vi "NetDifference.vi"() -> ()   [LabVIEW 2020]
uses:
  Globals and TypeDefs/Type Definitions.llb/FilePathParameter.ctt
  File and save/X-Axis_Generator_morph.vi
panel:
  out "Exp Index":u32
  in  "AutoSaveData":bool
  in  "stop 2":bool
  in  "SetDirectory?":bool
  in  "FilePath_C":T1={"Filename Prefix"="MyData", "Extension"=enum."±Field", "Suffix"="", "Current Path"=path "/opticsdata/Users"}
  out "?":T2(graph)
  in  "Toggle Subtraction":enum16{"Positive", "Negative"}(ring)
  in  "stop":bool
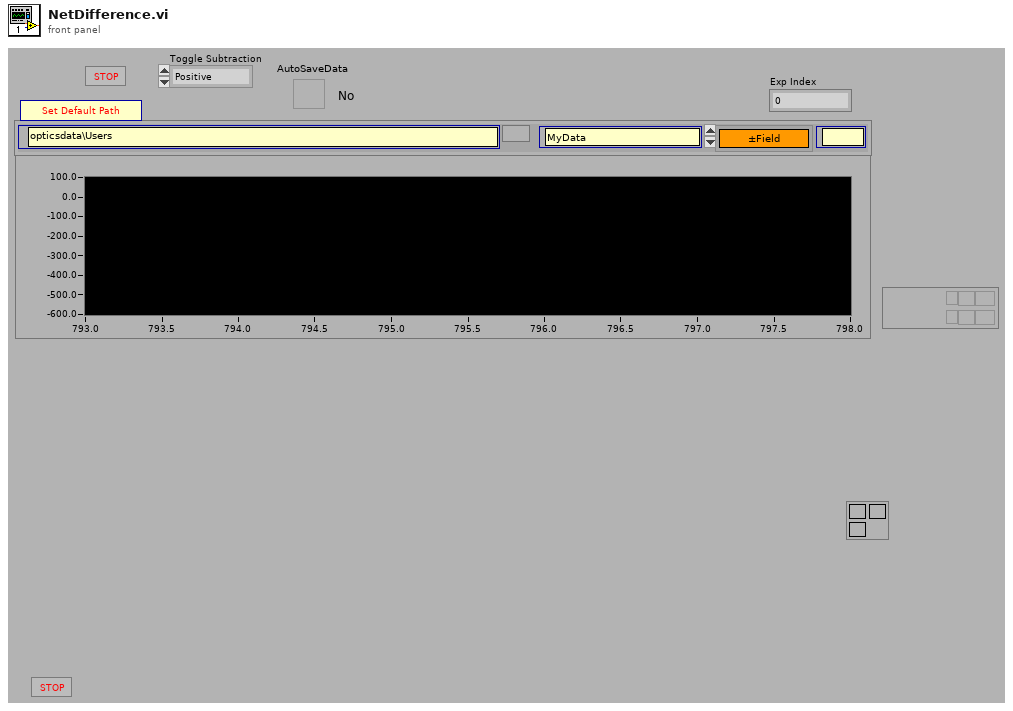
[diagram p1: front panel]
types:
  T1 = typedef "FilePathParameter.ctt" = cluster{"Filename Prefix":string, "Extension":enum16{"none", "\".001\",\".002\", ...", "001 (No dot)", "±Field", "pField nField", "Temperature", "Wavelength", "T(K)±H(T)", "(nm)T(K)±H(T)", "User Defined"}, "Suffix":string, "Current Path":path}
  T2 = cluster{"Ramp Pattern":dbl[], "Sinc Pattern":dbl[]}
  T3 = enum16{"Pass", "Write", "Read", "ReadPlotBlock", "Initialize", "InitFromBufferInput", "Resize Buffer"}
  T4 = enum16{"Auto Data Saving", "Manual Data Saving", "Auto Sequence Saving", "Sequence Saving from Data Buffer"}
  T5 = typedef "FileInfoParameter.ctt" = cluster{"FilePath":path, "Field (T)":dbl, "Temperature (K)":dbl, "X-Axis":T6, "Center nm":dbl, "Current Grating Density":T7, "CCD Parameters":T8, "Operation Mode":T9, "Exp Index":u32, "Index_repetition":u16, "Index":u16, "Current Detector":T10}
  T6 = typedef "Wavelength Unit.ctt" = enum8{"Point", "nm", "eV", "meV", "cm_1"}
  T7 = typedef "McPherson Grating Density.ctl" = enum8{"150", "300", "600", "1200", "1800"}
  T8 = typedef "CCDParameter.ctt" = cluster{"Exposure Time (s)":dbl, "Offset":dbl, "BkgrdCrct":bool, "Shutter":bool, "Mode":enum8{"Regular", "OverExp Cor", "SpikeRemove", "ForCalibration"}, "Repetition":u16, "dt or s":dbl}
  T9 = typedef "OperationMode.ctt" = enum16{"Standby", "CCD Single Shot", "CCD Sequence Shots", "CCD Custom Shots", "CCD Reference Shot", "Step Scanning ", "Time Scanning", "NML Data Acquisition"}
  T10 = typedef "ListOfDetectors.ctt" = enum8{"CCD-1024x256", "InGaAs PDA-1024x1", "CCD-1340x400", "Ge Single Channel", "Si Single Channel", "PMT Single Channel"}
  T11 = enum32{"existing file", "new file", "new or existing file", "existing dir", "new dir", "new or existing dir", "existing file (use LLBs)", "new file (use LLBs)", "new or existing file (use LLBs)", "new or existing file or directory (use LLBs)"}
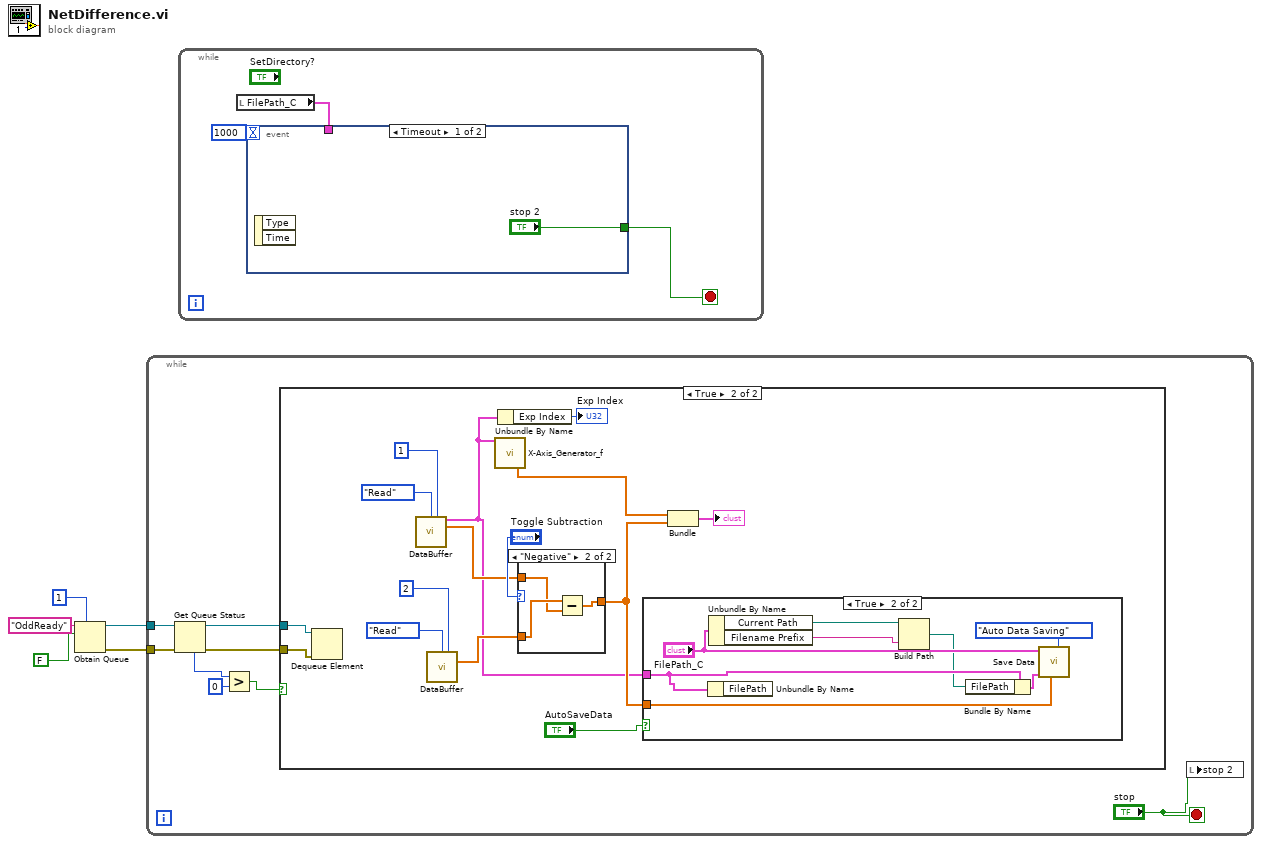
[diagram p0: block diagram]
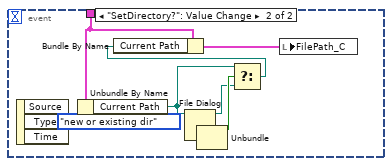
[diagram p2: hidden frame]
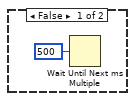
[diagram p3: hidden frame]
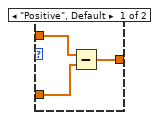
[diagram p5: hidden frame]
diagram:
  n1 = Obtain Queue(max queue size (-1, unlimited)=1, name (unnamed)="OddReady", element data type=FALSE ("Boolean")) -> (queue out=w3:refnum<queue>, error out=w2:errorcluster)  [unwired: 2 in, 1 out]
  n2 = while {
    tunnel: w3 -> [w13]
    tunnel: w2 -> [w12]
    stop <- "stop" stop-if-true
    n3 = Get Queue Status(queue=w13, error in (no error)=w12) -> (queue out=w7:refnum<queue>, error out=w8:errorcluster, # elements in queue=w10:i32)  [unwired: 1 in, 5 out]
    n4 = Greater?(x=w10, y=0) -> (0:w9:bool)
    n5 = case shown="True" w9 {
      tunnel: w8 -> [_ w19]
      tunnel: w7 -> [_ w18]
      frame False {
        n6 = Wait Until Next ms Multiple(millisecond multiple=u32 500 ("milliseconds to wait")) -> ()  [unwired: 1 out]
      }
      frame True {
        n7 = Dequeue Element(queue=w18, error in (no error)=w19) -> ()  [unwired: 1 in, 4 out]
        n8 = call "DataBuffer.vi"("Action"=T3."Read", "Read#"=1) -> ("File Info Out"=w16:T5, "Y Array out"=w23:dbl[])  [unwired: 9 in, 3 out]
        n9 = call "DataBuffer.vi"("Action"=T3."Read", "Read#"=2) -> ("Y Array out"=w24:dbl[])  [unwired: 9 in, 4 out]
        n10 = call-poly "X-Axis_Generator_f.vi"("File Info In"=w16) -> ("X-axis"=w22:dbl[])  [unwired: 11 in, 7 out]
        n11 = Unbundle By Name(w16) -> ("Exp Index"=→"Exp Index":u32)
        n12 = case shown="\"Negative\"" "Toggle Subtraction" {
          tunnel: w24 -> [w39 w43]
          tunnel: w23 -> [w40 w42]
          tunnel: [w38 w41] -> w20
          frame "Positive", Default {
            n13 = Subtract(x=w40, y=w39) -> (x-y=w38:dbl[])
          }
          frame "Negative" {
            n14 = Subtract(x=w43, y=w42) -> (x-y=w41:dbl[])
          }
        }
        n15 = case shown="True" "AutoSaveData" {
          tunnel: w16 -> [_ w33]
          tunnel: w20 -> [_ w37]
          frame False {
          }
          frame True {
            n16 = Unbundle By Name(w33) -> ()  [unwired: 1 out]
            n17 = Unbundle By Name("FilePath_C") -> ("Current Path"=w32:path, "Filename Prefix"=w31:string)
            n18 = Build Path(base path=w32, name or relative path=w31) -> (appended path=w30:path)
            n19 = Bundle By Name(cluster=w33, "FilePath"=w30) -> (w34:T5)
            n20 = call "Save Data.vi"("Saving Mode"=T4."Auto Data Saving", "Data"=w37, "File Info Input"=w34, "File Parameter"="FilePath_C") -> ()  [unwired: 7 in, 1 out]
          }
        }
        n21 = Bundle("X-axis"=w22, w20) -> (→"?":cluster{"X-axis":dbl[], dbl[]})  [unwired: 1 in]
      }
    }
    n22 = local write "stop 2"("stop") -> ()
  }
  n23 = while {
    stop <- w45 stop-if-true
    n24 = local read "FilePath_C"() -> (w46:T1)
    n25 = event shown="[0] Timeout" {
      selector: _ -> [_ _]
      dyn-events: _ -> [_ _]
      timeout: 1000 -> [_ _]
      tunnel: w46 -> [_ w52]
      tunnel: ["stop 2" _] -> w45
      event Timeout {
        n26 = event-data() -> ()  [unwired: 1 in, 2 out]
      }
      event "SetDirectory?": Value Change {
        (unwired) T11."new or existing dir" ("select mode (2)")
        n27 = event-data() -> ()  [unwired: 1 in, 3 out]
        n28 = Unbundle By Name(w52) -> ("Current Path"=w53:path)
        n29 = File Dialog(11:w53) -> (0:w48:errorcluster, 1:w51:bool, 3:w50:path)  [unwired: 6 in, 1 out]
        n30 = Unbundle(w48) -> ()  [unwired: 3 out]
        n31 = Select(t=w53, s=w51, f=w50) -> (s? t:f=w54:path)
        n32 = Bundle By Name(cluster=w52, "Current Path"=w54) -> (w49:T1)
        n33 = local write "FilePath_C"(w49) -> ()
      }
    }
  }
